vi "Main.vi"() -> ()   [LabVIEW 2020]
uses:
  Tread.lvclass
panel:
  out "error out":errorcluster
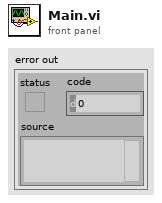
[diagram p1: front panel]
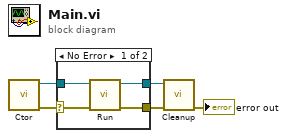
[diagram p0: block diagram]
diagram:
  n1 = call "Ctor.vi"() -> ("error out"=w5:errorcluster, "Tread out"=w4:refnum<class "Tread.lvclass">)  [unwired: 10 in]
  n2 = case shown="No Error" w5 {
    selector: w5 -> [w8 w10]
    tunnel: w4 -> [w9 w11]
    tunnel: [w7 w11] -> w3
    tunnel: [w6 w10] -> w2
    frame No Error {
      n3 = call "Run.vi"("error in (no error)"=w8, "Tread in"=w9) -> ("error out"=w6:errorcluster, "Tread out"=w7:refnum<class "Tread.lvclass">)  [unwired: 8 in]
    }
    frame Error {
    }
  }
  n4 = call "Cleanup.vi"("error in (no error)"=w2, "Tread in"=w3) -> ("error out"=→"error out":errorcluster)  [unwired: 9 in]
